vi "Regatron.G5.Rest VoltageSampleSmall.vi"() -> ()   [LabVIEW 2021, in "G5 Regatron Custom Device Shared.lvlib"]
uses:
  G5 Regatron Custom Device/Shared/G5 Regatron Custom Device Shared.lvlib
  Regatron.G5.Rest Handle.llb/G5.Rest Status.ctl
  Regatron.G5.Rest System.llb/G5.Rest System Output References.ctl
  Regatron.G5.Rest System.llb/G5.Rest System Output References Datasource.ctl
  Regatron.G5.Rest System.llb/G5.Rest System Output Limits Datasource.ctl
  Regatron.G5.Rest System.llb/G5.Rest System Output Limits.ctl
  <vilib>/Addons/_JKI.lib/REST Client/classes/REST Client/REST Client.lvclass
  Regatron.G5.Rest.lvlib
panel:
  in  "VOLTAGE ON/OFF":bool
  out "Voltage actual state":bool
  out "State":string
  in  "stop vi execution":bool
  in  "IP":string="192.168.1.210"
  in  "V":dbl min=0.0 max=500.0 step=0.125 format="%.2f"
  out "Output Voltage":string
  out "error out":errorcluster
  in  "error in (no error)":errorcluster
  # "Output Voltage"
  # "Voltage Preset"
  # "V"
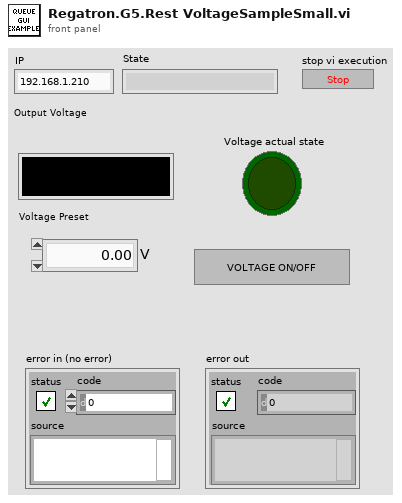
[diagram p1: front panel]
types:
  T1 = typedef "G5 Regatron Custom Device Shared.lvlib/Regatron.G5.Rest.lvlib/G5.Rest Status.ctl" = enum16{"Read", "Write"}
  T2 = typedef "G5 Regatron Custom Device Shared.lvlib/Regatron.G5.Rest.lvlib/G5.Rest System Output Limits.ctl" = cluster{"Voltage Upper Limit V":sgl, "Voltage Lower Limit V":sgl, "Current Upper Limit A":sgl, "Current Lower Limit A":sgl, "Power Upper Limit W":sgl, "Power Lower Limit W":sgl}
  T3 = typedef "G5 Regatron Custom Device Shared.lvlib/Regatron.G5.Rest.lvlib/G5.Rest System Output References.ctl" = cluster{"Voltage V":sgl, "Current A":sgl, "Power W":sgl, "Load R Ohm":sgl}
  T4 = typedef "G5 Regatron Custom Device Shared.lvlib/Regatron.G5.Rest.lvlib/G5.Rest System Output Values.ctl" = cluster{"Voltage V":sgl, "Current A":sgl, "Power W":sgl, "Power kW":sgl, "Load R Ohm":sgl}
  T5 = typedef "G5 Regatron Custom Device Shared.lvlib/Regatron.G5.Rest.lvlib/G5.Rest System Output Limits Datasource.ctl" = enum16{"Voltage Upper Limit", "Voltage Lower Limit", "Current Upper Limit", "Current Lower Limit", "Power Upper Limit", "Power Lower Limit", "ALL"}[]
  T6 = typedef "G5 Regatron Custom Device Shared.lvlib/Regatron.G5.Rest.lvlib/G5.Rest System Output References Datasource.ctl" = enum16{"Voltage", "Current", "Power", "Load Resistance", "ALL"}[]
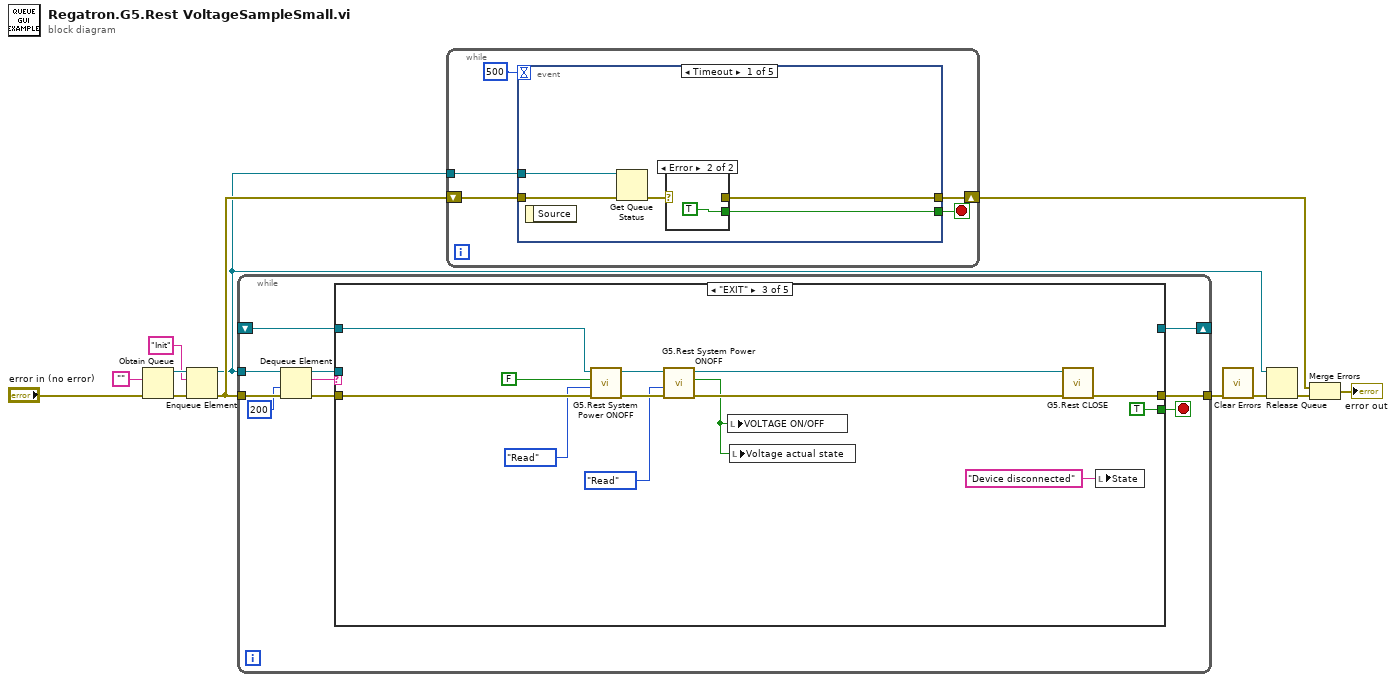
[diagram p0: block diagram]
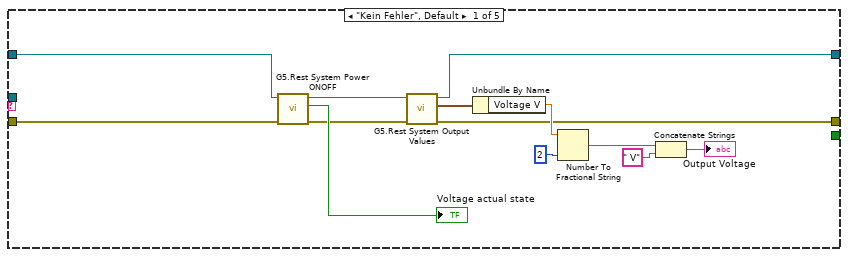
[diagram p2: hidden frame]
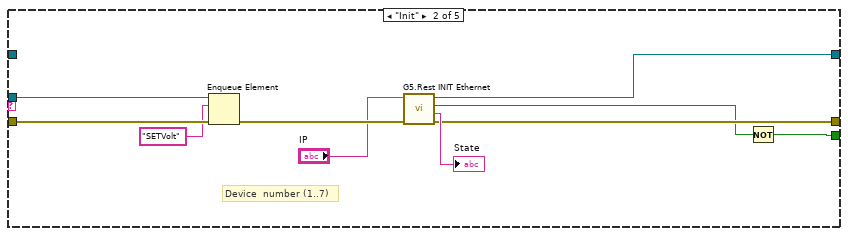
[diagram p3: hidden frame]
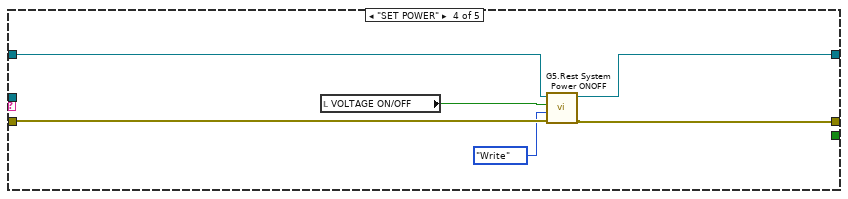
[diagram p4: hidden frame]
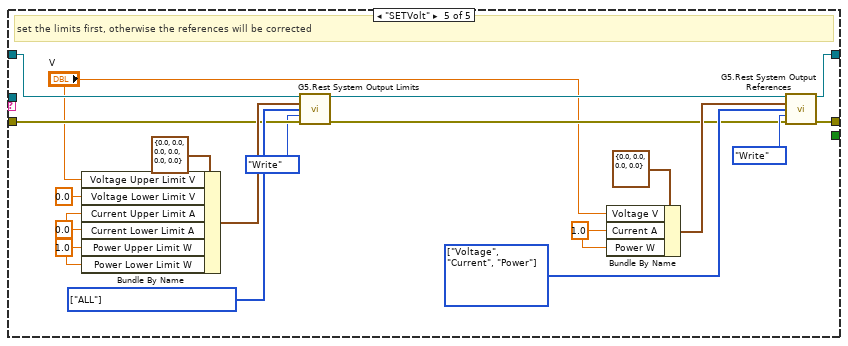
[diagram p5: hidden frame]
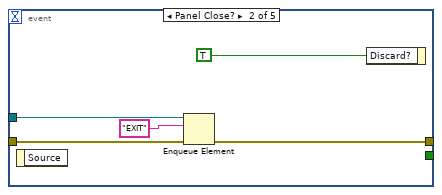
[diagram p7: hidden frame]
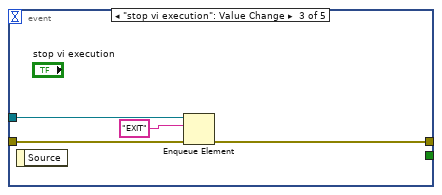
[diagram p8: hidden frame]
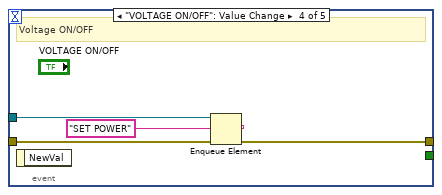
[diagram p9: hidden frame]
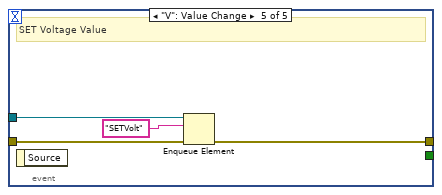
[diagram p10: hidden frame]
diagram:
  n1 = Obtain Queue(element data type="", error in (no error)="error in (no error)") -> (queue out=w10:refnum<queue>, error out=w11:errorcluster)  [unwired: 3 in, 1 out]
  n2 = Enqueue Element(queue=w10, element="Init" ("Element"), error in (no error)=w11) -> (queue out=w5:refnum<queue>, error out=w9:errorcluster)  [unwired: 1 in, 1 out]
  n3 = while {
    tunnel: w5 -> [w22]
    tunnel: w9 -> [w19]
    tunnel: [w17] -> w1
    shift-right: [w14] -> _
    shift-left: _ -> [w13]
    stop <- w21 stop-if-true
    n4 = Dequeue Element(queue=w22, timeout in ms (-1)=200 ("Timeout in ms (-1)"), error in (no error)=w19) -> (queue out=w15:refnum<queue>, element=w20:string, error out=w18:errorcluster)  [unwired: 1 out]
    n5 = case shown="\"EXIT\"" w20 {
      tunnel: [_ w45 TRUE _ _] -> w21
      tunnel: w18 -> [w30 w44 w55 w63 w70]
      tunnel: [w27 w40 w49 w64 w78] -> w17
      tunnel: w15 -> [_ w43 _ _ _]
      tunnel: [w24 w37 _ w61 w77] -> w14
      tunnel: w13 -> [w29 _ w51 w62 w69]
      frame "Kein Fehler", Default {
        n6 = call "G5.Rest System Power ONOFF.vi"("Fehler (Eingang, kein Fehler)"=w30, "G5 WEB API (Eingang)"=w29) -> ("Fehler (Ausgang)"=w26:errorcluster, "Get Power OFF/ON"=→"Voltage actual state":bool, "G5 WEB API (Ausgang)"=w25:refnum<class "REST Client.lvclass">)  [unwired: 7 in]
        n7 = call "G5.Rest System Output Values.vi"("Fehler (Eingang, kein Fehler)"=w26, "G5 WEB API (Eingang)"=w25) -> ("Fehler (Ausgang)"=w27:errorcluster, "Output Values"=w23:T4, "G5 WEB API (Ausgang)"=w24:refnum<class "REST Client.lvclass">)  [unwired: 7 in]
        n8 = Unbundle By Name(w23) -> ("Voltage V"=w31:sgl)
        n9 = Number To Fractional String(number=w31, precision (6)=i16 2) -> (F-format string=w35:string)  [unwired: 2 in]
        n10 = Concatenate Strings(w35, " V" ("string")) -> (→"Output Voltage":string)
      }
      frame "Init" {
        # "Device  number (1..7)"
        n11 = Enqueue Element(queue=w43, element="SETVolt" ("Element"), error in (no error)=w44) -> (error out=w39:errorcluster)  [unwired: 1 in, 2 out]
        n12 = call "G5.Rest INIT Ethernet.vi"("error in (no error)"=w39, "IP"="IP") -> ("error out"=w40:errorcluster, "State"=→"State":string, "Device found"=w38:bool, "G5 WEB API"=w37:refnum<class "REST Client.lvclass">)  [unwired: 5 in, 1 out]
        n13 = Not(x=w38) -> (.not. x?=w45:bool)
      }
      frame "EXIT" {
        n14 = call "G5.Rest System Power ONOFF.vi"("Fehler (Eingang, kein Fehler)"=w55, "Status"=G5.Rest_Status."Read", "Power OFF/ON"=FALSE ("TC Actual State SET"), "G5 WEB API (Eingang)"=w51) -> ("Fehler (Ausgang)"=w56:errorcluster, "G5 WEB API (Ausgang)"=w50:refnum<class "REST Client.lvclass">)  [unwired: 5 in, 1 out]
        n15 = call "G5.Rest System Power ONOFF.vi"("Fehler (Eingang, kein Fehler)"=w56, "Status"=G5.Rest_Status."Read", "G5 WEB API (Eingang)"=w50) -> ("Fehler (Ausgang)"=w48:errorcluster, "Get Power OFF/ON"=w46:bool, "G5 WEB API (Ausgang)"=w47:refnum<class "REST Client.lvclass">)  [unwired: 6 in]
        n16 = local write "VOLTAGE ON/OFF"(w46) -> ()
        n17 = local write "Voltage actual state"(w46) -> ()
        n18 = call "G5.Rest CLOSE.vi"("Fehler (Eingang, kein Fehler)"=w48, "G5 WEB API"=w47) -> ("error out"=w49:errorcluster)  [unwired: 9 in]
        n19 = local write "State"("Device disconnected" ("State")) -> ()
      }
      frame "SET POWER" {
        n20 = local read "VOLTAGE ON/OFF"() -> (w60:bool)
        n21 = call "G5.Rest System Power ONOFF.vi"("Fehler (Eingang, kein Fehler)"=w63, "Status"=G5.Rest_Status."Write", "Power OFF/ON"=w60, "G5 WEB API (Eingang)"=w62) -> ("Fehler (Ausgang)"=w64:errorcluster, "G5 WEB API (Ausgang)"=w61:refnum<class "REST Client.lvclass">)  [unwired: 5 in, 1 out]
      }
      frame "SETVolt" {
        w72 = sgl 0.0 ("Current Lower Limit A")
        w73 = sgl 1.0 ("Power Upper Limit W")
        w71 = T5 [enum."ALL"] items=["Voltage Upper Limit", "Voltage Lower Limit", "Current Upper Limit", "Current Lower Limit", "Power Upper Limit", "Power Lower Limit", "ALL"] ("Datasource")
        w79 = T6 [enum."Voltage", enum."Current", enum."Power"] items=["Voltage", "Current", "Power", "Load Resistance", "ALL"] ("Datasource")
        w83 = 1.0 ("Current Q1 A")
        # "set the limits first, otherwise the references will be corrected"
        n22 = Bundle By Name(cluster=T2 {"Voltage Upper Limit V"=0.0, "Voltage Lower Limit V"=0.0, "Current Upper Limit A"=0.0, "Current Lower Limit A"=0.0, "Power Upper Limit W"=0.0, "Power Lower Limit W"=0.0} ("SET Output Limit"), "Voltage Upper Limit V"="V", "Voltage Lower Limit V"=sgl 0.0, "Current Upper Limit A"=w73, "Current Lower Limit A"=w72, "Power Upper Limit W"=w73, "Power Lower Limit W"=w72) -> (w76:T2)
        n23 = call "G5.Rest System Output Limits.vi"("G5 WEB API (Eingang)"=w69, "SET Output Limit"=w76, "Datasource"=w71, "Status"=G5.Rest_Status."Write", "Fehler (Eingang, kein Fehler)"=w70) -> ("G5 WEB API (Ausgang)"=w67:refnum<class "REST Client.lvclass">, "Fehler (Ausgang)"=w68:errorcluster)  [unwired: 8 in, 1 out]
        n24 = Bundle By Name(cluster=T3 {"Voltage V"=0.0, "Current A"=0.0, "Power W"=0.0, "Load R Ohm"=0.0} ("SET Output Reference"), "Voltage V"="V", "Current A"=w83, "Power W"=w83) -> (w81:T3)
        n25 = call "G5.Rest System Output References .vi"("G5 WEB API (Eingang)"=w67, "SET Output Reference"=w81, "Datasource"=w79, "Status"=G5.Rest_Status."Write", "Fehler (Eingang, kein Fehler)"=w68) -> ("G5 WEB API (Ausgang)"=w77:refnum<class "REST Client.lvclass">, "Fehler (Ausgang)"=w78:errorcluster)  [unwired: 8 in, 1 out]
      }
    }
  }
  n26 = while {
    shift-right: [w86] -> w8
    shift-left: w9 -> [w87]
    tunnel: w5 -> [w88]
    stop <- w84 stop-if-true
    n27 = event "Ereignisstruktur" shown="[0] Timeout" {
      selector: _ -> [_ _ _ _ _]
      dyn-events: _ -> [_ _ _ _ _]
      timeout: 500 -> [_ _ _ _ _]
      tunnel: w88 -> [w92 w97 w102 w107 w111]
      tunnel: w87 -> [w93 w98 w103 w108 w112]
      tunnel: [w90 w96 w101 w106 w110] -> w86
      tunnel: [w89 _ _ _ _] -> w84
      event Timeout {
        n28 = event-data() -> ()  [unwired: 1 in, 1 out]
        n29 = Get Queue Status(queue=w92, error in (no error)=w93) -> (error out=w91:errorcluster)  [unwired: 1 in, 7 out]
        n30 = case shown="Error" w91 {
          selector: w91 -> [w94 _]
          tunnel: [w94 _] -> w90
          tunnel: [_ TRUE] -> w89
          frame No Error {
          }
          frame Error {
          }
        }
      }
      event Panel Close? {
        n31 = event-data() -> ()  [unwired: 1 in, 1 out]
        n32 = Enqueue Element(queue=w97, element="EXIT", error in (no error)=w98) -> (error out=w96:errorcluster)  [unwired: 1 in, 2 out]
        n33 = event-data("Discard?"=TRUE) -> ()  [unwired: 1 in, 1 out]
      }
      event "stop vi execution": Value Change {
        n34 = event-data() -> ()  [unwired: 1 in, 1 out]
        n35 = Enqueue Element(queue=w102, element="EXIT", error in (no error)=w103) -> (error out=w101:errorcluster)  [unwired: 1 in, 2 out]
      }
      event "VOLTAGE ON/OFF": Value Change {
        # "Voltage ON/OFF"
        n36 = event-data() -> ()  [unwired: 1 in, 1 out]
        n37 = Enqueue Element(queue=w107, element="SET POWER" ("Element"), error in (no error)=w108) -> (error out=w106:errorcluster)  [unwired: 1 in, 2 out]
      }
      event "V": Value Change {
        # "SET Voltage Value"
        n38 = event-data() -> ()  [unwired: 1 in, 1 out]
        n39 = Enqueue Element(queue=w111, element="SETVolt" ("Element"), error in (no error)=w112) -> (error out=w110:errorcluster)  [unwired: 1 in, 2 out]
      }
    }
  }
  n40 = call <vilib>:"Clear Errors.vi"("error in (no error)"=w1) -> ("error out"=w2:errorcluster)  [unwired: 5 in, 1 out]
  n41 = Release Queue(queue=w5, error in (no error)=w2) -> (error out=w4:errorcluster)  [unwired: 1 in, 2 out]
  n42 = Merge Errors(w8, w4) -> (→"error out":errorcluster)
